vi "Set Struct Transfer Mode.vi"(8 "error in":errorcluster, 10 "Allow struct tranfer (False)":bool, 11 "GOLPI ref. in":T1={"pipe handle"={"lv_proc.dll file path"=path "", "process instance handle"=[], "debug mode"=FALSE, "debug data"=[]}, "fast read timeout [ms]"=500, "fast read settle time [ms]"=10, "fast read to multiple [ms]"=1, "max elements per input line"=100, "slow read timeout [ms]"=5000, "stdin double format specifier"="", "max elements per stdout output column"=100, "console mode bitstream"=FALSE, "bitstream first read timeout [ms]"=1000, "bitstream read timeout [ms]"=50, "struct transfer possible"=FALSE, "matlab mode"=FALSE}) -> (0 "error out":errorcluster, 2 "conv struct possible?":bool, 3 "GOLPI ref. out":T1={"pipe handle"={"lv_proc.dll file path"=path "", "process instance handle"=[], "debug mode"=FALSE, "debug data"=[]}, "fast read timeout [ms]"=500, "fast read settle time [ms]"=10, "fast read to multiple [ms]"=1, "max elements per input line"=100, "slow read timeout [ms]"=5000, "stdin double format specifier"="", "max elements per stdout output column"=100, "console mode bitstream"=FALSE, "bitstream first read timeout [ms]"=1000, "bitstream read timeout [ms]"=50, "struct transfer possible"=FALSE, "matlab mode"=FALSE})   [LabVIEW 2020, in "GOLPI library.lvlib"]
doc: "Set structure transfer mode (GNU Octave mode only, not allowed in Matlab mode). This is required for transfering of GNU Octave structures into LabVIEW cluster. First this VI tries to install GNU Octave package golpi. Than package is loaded and VI checks if function golpi_conv_struct() is available in current GNU Octave instance. If not the VIs related to structure tranfer will generate errors. This VI must be called before the structure transfer VIs can be used.\n\n---\nGOLPI works only with lv_proc.dll library, which is part of vipm package or should be delivered together with packed library. Placement of this dll is selected in terminal of Start GNU Octave.vi."
uses:
  GOLPI library.lvlib
  GOLPI reference Type Def.ctl
  Pipe Handle.ctl
  Custom Error Codes Enum Type Def.vi
  <vilib>/regexp/Match Regular Expression.xnode
  LV Process library.lvlib
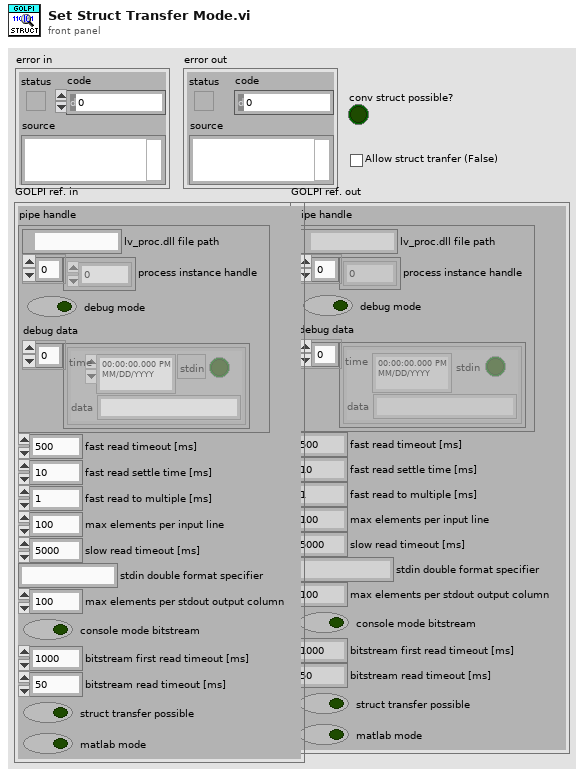
[diagram p1: front panel]
types:
  T1 = typedef "GOLPI library.lvlib/GOLPI reference Type Def.ctl" = cluster{"pipe handle":T2, "fast read timeout [ms]":u32, "fast read settle time [ms]":u32, "fast read to multiple [ms]":u32, "max elements per input line":u32, "slow read timeout [ms]":u32, "stdin double format specifier":string, "max elements per stdout output column":u32, "console mode bitstream":bool, "bitstream first read timeout [ms]":u32, "bitstream read timeout [ms]":u32, "struct transfer possible":bool, "matlab mode":bool}
  T2 = typedef "LV Process library.lvlib/Pipe Handle.ctl" = cluster{"lv_proc.dll file path":path, "process instance handle":u32[], "debug mode":bool, "debug data":cluster{"time":timestamp, "stdin":bool, "data":string}[]}
  T3 = typedef "GOLPI library.lvlib/Custom Error Codes Enum Type Def.vi" = enum16{"no error", "00 working directory PAR1 missing", "01 octave binary PAR1 missing", "02 octave report error PAR1", "03 empty output last cmd PAR1", "04 missing temporary file PAR1", "05 pwd PAR 1 not exist", "06 oct package not installed", "07 octave default binary missing", "10 var PAR1 not string, vect", "11 var PAR1 not num, scal, ~compl", "12 var PAR1 not num, scal, compl", "13 var PAR1 not num, vect, ~compl", "14 var PAR1 not num, vect, compl", "15 var PAR1 not num, mat, ~compl", "16 var PAR1 not num, mat, ~compl", "30 read timeout", "60 bitstream transport failed", "61 bitstream decode error PAR1", "62 bitstream cannot be set", "70 struct transfer not possible", "80 struct: cluster elem. PAR1 not implem.", "81 struct: structure field PAR1 not implem.", "82 struct: size mismatch of PAR1", "83 struct: type mismatch of PAR1", "98 internal error", "99 not finished", "90 Not supported in Matlab mode", "91 Matlab variable transfer error", "92 Matlab Script Error"}
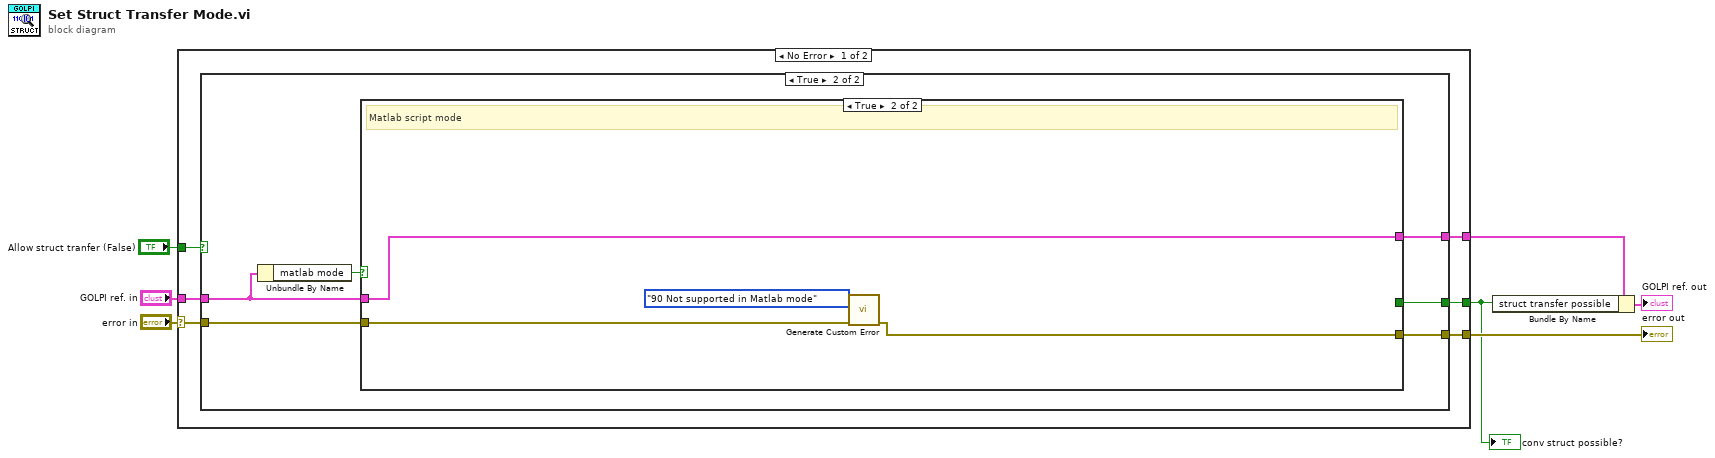
[diagram p0: block diagram]
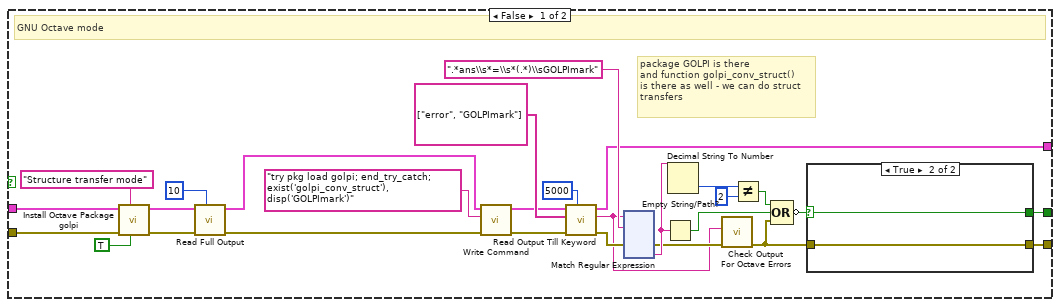
[diagram p3: hidden frame]
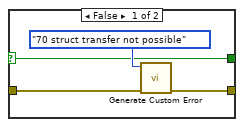
[diagram p4: hidden frame]
diagram:
  n1 = case shown="No Error" "error in" {
    selector: "error in" -> [w13 w177]
    tunnel: "GOLPI ref. in" -> [w8 w176]
    tunnel: [w12 w177] -> w5
    tunnel: [w11 w176] -> w3
    tunnel: [w10 _] -> w2
    tunnel: "Allow struct tranfer (False)" -> [w9 _]
    frame No Error {
      n2 = case shown="True" w9 {
        tunnel: w8 -> [w14 w17]
        tunnel: w13 -> [w15 w18]
        tunnel: [w15 w20] -> w12
        tunnel: [w14 w21] -> w11
        tunnel: [_ w19] -> w10
        frame False {
        }
        frame True {
          n3 = Unbundle By Name(w17) -> ("matlab mode"=w16:bool)
          n4 = case shown="True" w16 {
            tunnel: [w32 w173] -> w21
            tunnel: [w30 w174] -> w20
            tunnel: [w28 _] -> w19
            tunnel: w17 -> [w25 w173]
            tunnel: w18 -> [w24 w175]
            frame False {
              # "package GOLPI is there\nand function golpi_conv_struct()\nis there as well - we can do struct\ntransfers"
              # "GNU Octave mode"
              n5 = call "Install Octave Package golpi.vi"("Verbose? (T)"=TRUE, "Feature name"="Structure transfer mode", "error in"=w24, "GOLPI ref. in"=w25) -> ("error out"=w23:errorcluster, "GOLPI ref. out"=w22:T1)  [unwired: 6 in]
              n6 = call "Read Full Output.vi"("timeout [ms]"=u32 10, "error in"=w23, "GOLPI ref. in"=w22) -> ("error out"=w48:errorcluster, "GOLPI ref. out"=w49:T1)  [unwired: 5 in, 2 out]
              n7 = call "Write Command.vi"("error in"=w48, "command"="try pkg load golpi; end_try_catch; exist('golpi_conv_struct'), disp('GOLPImark')", "GOLPI ref. in"=w49) -> ("error out"=w39:errorcluster, "GOLPI ref. out"=w37:T1)  [unwired: 7 in]
              n8 = call "Read Output Till Keyword.vi"("timeout [ms]"=u32 5000, "error in"=w39, "keywords"=string[] ["error", "GOLPImark"], "GOLPI ref. in"=w37) -> ("error out"=w38:errorcluster, "read buffer"=w33:string, "GOLPI ref. out"=w32:T1)  [unwired: 4 in, 1 out]
              n9 = xnode "Match Regular Expression"("input string"=w33, "regular expression"=".*ans\\s*=\\s*(.*)\\sGOLPImark", "error in"=w38) -> ("error out"=w40:errorcluster, "submatch 1"=w43:string)  [unwired: 3 in, 4 out]
              n10 = Empty String/Path?(string/path=w43) -> (empty?=w44:bool)
              n11 = Decimal String To Number(string=w43) -> (number=w34:i32)  [unwired: 2 in, 1 out]
              n12 = call "Check Output For Octave Errors.vi"("error in"=w40, "read buffer"=w33) -> ("error out"=w31:errorcluster)  [unwired: 9 in]
              n13 = Not Equal?(x=w34, y=2) -> (x != y?=w41:bool)
              n14 = Compound Arithmetic op=OR(w41, w44, w31) -> (invert w29:bool)
              n15 = case shown="True" w29 {
                selector: w29 -> [w50 w54]
                tunnel: w31 -> [w53 w55]
                tunnel: [w52 w55] -> w30
                tunnel: [w50 w54] -> w28
                frame False {
                  n16 = call "Generate Custom Error.vi"("error in"=w53, "GOLPI error"=Custom_Error_Codes_Enum_Type_Def.vi."70 struct transfer not possible") -> ("error out"=w52:errorcluster)  [unwired: 9 in]
                }
                frame True {
                }
              }
            }
            frame True {
              # "Matlab script mode"
              n17 = call "Generate Custom Error.vi"("error in"=w175, "GOLPI error"=Custom_Error_Codes_Enum_Type_Def.vi."90 Not supported in Matlab mode") -> ("error out"=w174:errorcluster)  [unwired: 9 in]
            }
          }
        }
      }
    }
    frame Error {
    }
  }
  "error out" <- w5
  "conv struct possible?" <- w2
  n18 = Bundle By Name(cluster=w3, "struct transfer possible"=w2) -> (→"GOLPI ref. out":T1)
